vi "ConfigureCurrent.vi"(8 "error in (no error)":errorcluster, 10 "Current(0)":dbl, 11 "YP03-60_Z in":refnum<class "YP03-60_Z.lvclass">) -> (0 "error out":errorcluster, 3 "YP03-60_Z out":refnum<class "YP03-60_Z.lvclass">)   [LabVIEW 2020, in "PowerControl.lvlib" / "YP03-60_Z.lvclass"]
uses:
  YP03-60_Z.lvclass
  YP03-60_Z.lvclass/YP03-60_Z.ctl
  <vilib>/Instr/_visa.llb/VISA Configure Serial Port (Instr).vi
  VirtualPower/VirtualPower.lvclass
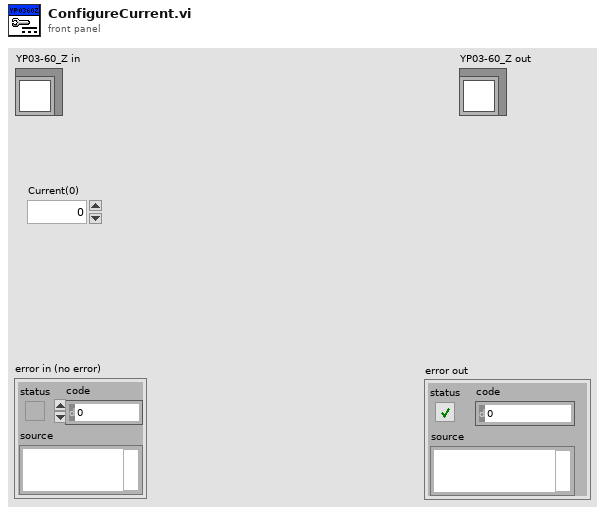
[diagram p1: front panel]
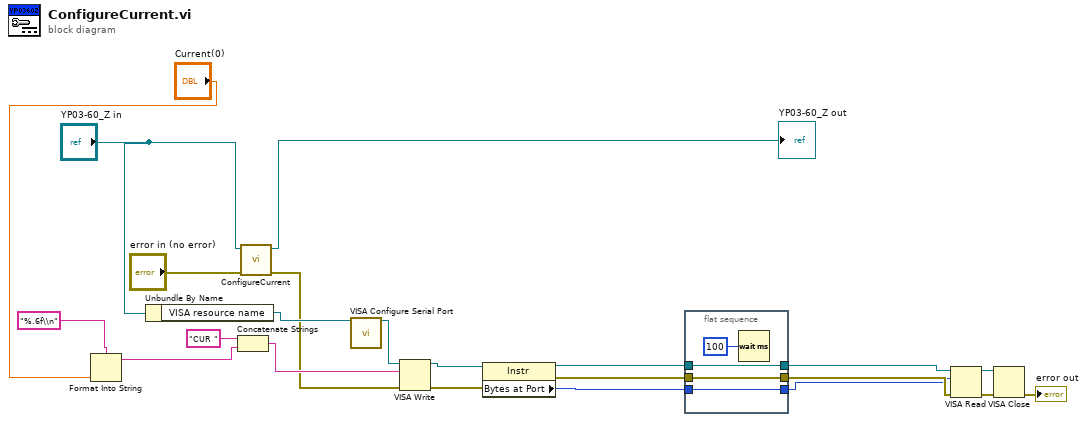
[diagram p0: block diagram]
diagram:
  n1 = Format Into String(format string="%.6f\\n", "Current(0)") -> (resulting string=w16:string)  [unwired: 2 in, 1 out]
  n2 = Unbundle By Name("YP03-60_Z in") -> ("VISA resource name"=w19:refnum<visa-resource-name>)
  n3 = Concatenate Strings("CUR " ("string"), w16) -> (w14:string)
  n4 = call-parent "ConfigureCurrent.vi"("error in (no error)"="error in (no error)", "VirtualPower in"="YP03-60_Z in") -> ("error out"=w1:errorcluster, "VirtualPower out"=→"YP03-60_Z out":refnum<class "YP03-60_Z.lvclass">)  [unwired: 8 in]
  n5 = call-poly "VISA Configure Serial Port"("VISA resource name"=w19) -> ("VISA resource name out"=w13:refnum<visa-resource-name>)  [unwired: 13 in, 1 out]
  n6 = VISA Write(VISA resource name=w13, write buffer=w14, error in (no error)=w1) -> (VISA resource name out=w12:refnum<visa-resource-name>, error out=w11:errorcluster)  [unwired: 1 out]
  n7 = property class="Instr"(reference=w12, error in=w11) -> (reference out=w6:refnum<visa-resource-name>, error out=w5:errorcluster, "Bytes at Port"=w4:u32)
  n8 = flat-sequence {
    tunnel: w6 -> [w26]
    tunnel: [w26] -> w10
    tunnel: [w25] -> w2
    tunnel: w4 -> [w25]
    tunnel: [w24] -> w3
    tunnel: w5 -> [w24]
    frame #0 {
      n9 = Wait (ms)(milliseconds to wait=u32 100) -> ()  [unwired: 1 out]
    }
  }
  n10 = VISA Read(VISA resource name=w10, byte count=w2, error in (no error)=w3) -> (VISA resource name out=w9:refnum<visa-resource-name>, error out=w7:errorcluster)  [unwired: 2 out]
  n11 = VISA Close(VISA resource name=w9, error in (no error)=w7) -> (error out=→"error out":errorcluster)
